vi "BasicExample.vi"() -> ()   [LabVIEW 2019]
panel:
  in  "stop":bool
  out "element":string
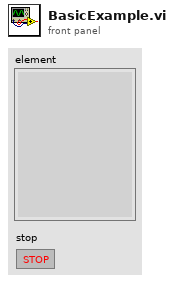
[diagram p1: front panel]
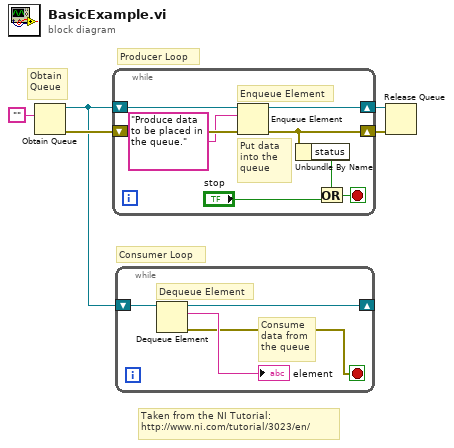
[diagram p0: block diagram]
diagram:
  # "Taken from the NI Tutorial:\nhttp://www.ni.com/tutorial/3023/en/"
  # "Consumer Loop"
  # "Obtain\nQueue"
  # "Producer Loop"
  n1 = Obtain Queue(element data type="") -> (queue out=w3:refnum<queue>, error out=w4:errorcluster)  [unwired: 4 in, 1 out]
  n2 = while {
    shift-right: [w10] -> w1
    shift-left: w4 -> [w13]
    shift-right: [w6] -> w2
    shift-left: w3 -> [w11]
    stop <- w8 stop-if-true
    # "Put data into the queue"
    # "Enqueue Element"
    n3 = Enqueue Element(queue=w11, element="Produce data to be placed in the queue.", error in (no error)=w13) -> (queue out=w6:refnum<queue>, error out=w10:errorcluster)  [unwired: 1 in, 1 out]
    n4 = Unbundle By Name(w10) -> ("status"=w9:bool)
    n5 = Or(x=w9, y="stop") -> (x .or. y?=w8:bool)
  }
  n6 = while {
    shift-right: [w14] -> _
    shift-left: w3 -> [w17]
    stop <- w15 stop-if-true
    # "Consume data from the queue"
    # "Dequeue Element"
    n7 = Dequeue Element(queue=w17) -> (queue out=w14:refnum<queue>, element=→"element":string, error out=w15:errorcluster)  [unwired: 2 in, 1 out]
  }
  n8 = Release Queue(queue=w2, error in (no error)=w1) -> ()  [unwired: 1 in, 3 out]
